vi "Camera Stream Properties.vi"() -> ()   [LabVIEW 2014]
doc: "When a camera stream is successfully opened, it is possible to edit its properties, like resolution and brightness.\nPlease note that the available properties are dependent on the camera type and driver."
uses:
  MSC Video_class/controls/Stream Property.ctl
  MSC Video_class/MSC Video.lvclass
  MSC Image_class/MSC Image.lvclass
panel:
  in  "Set":bool
  in  "New Value":dbl format="%#_3f"
  in  "Property":T1=3 caption="Camera Stream Property" items=["Position msec", "Position frames", "Position avi ratio", "Frame Width", "Frame Height", "FPS", "FourCC codec", "Frame Count", "Format", "Mode", "Brightness", "Contrast", "Saturation", "Hue", "Gain", "Exposure", "Convert RGB", "White Balance U", "Rectification", "Monochrome", "Sharpness", "Auto Exposure", "Gamma", "Temperature", "Trigger", "Trigger Delay", "White Balance V", "Zoom", "Focus", "Guid", "ISO Speed", "Max DV1394", "Backlight", "Pan", "Tilt", "Rolls", "Iris", "Settings", "Buffersize"]
  out "Properties":string[][](array[string])
  out "error out":errorcluster
  in  "stop":bool
  out "Live Image":picture
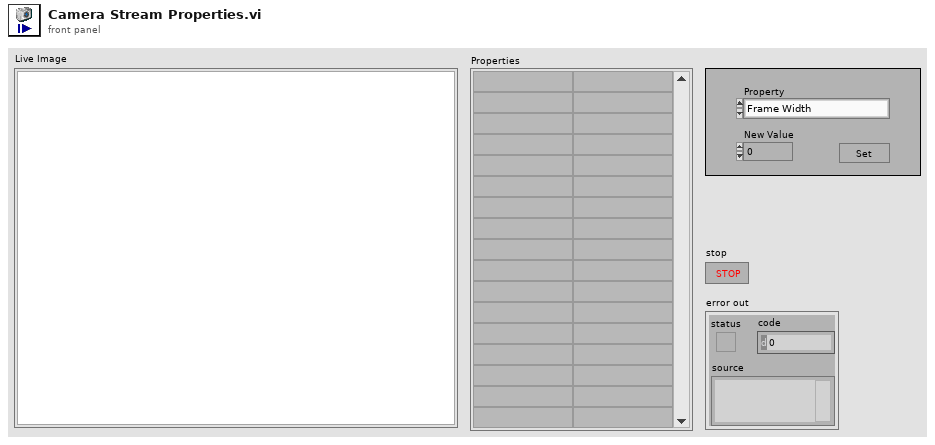
[diagram p1: front panel]
types:
  T1 = typedef "MSC Video.lvclass/Stream Property.ctl" = u16
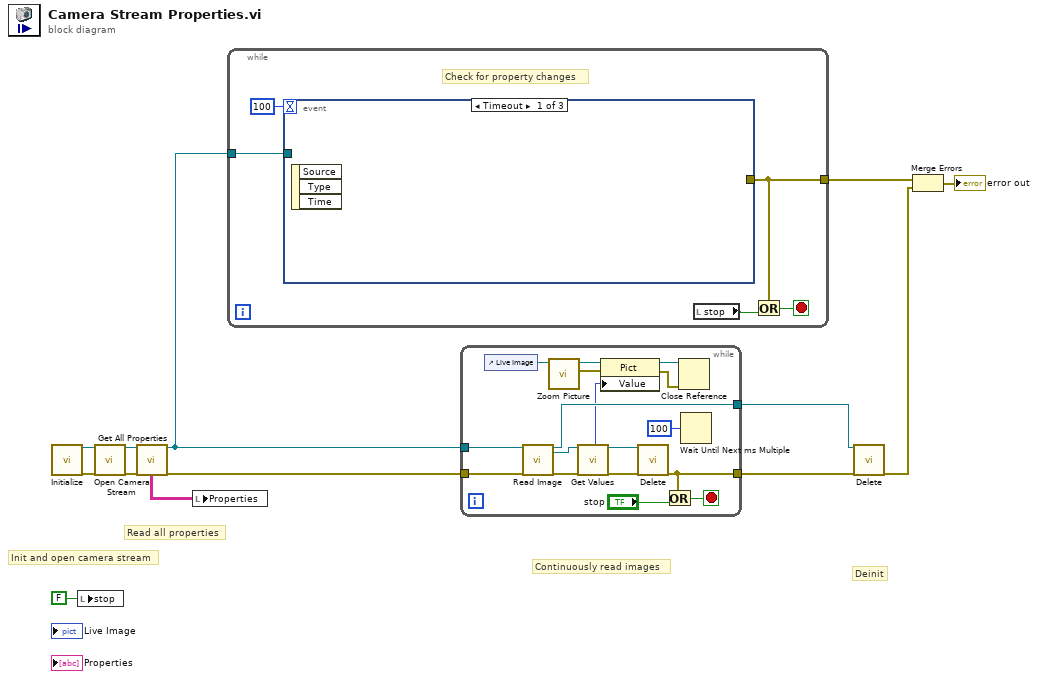
[diagram p0: block diagram]
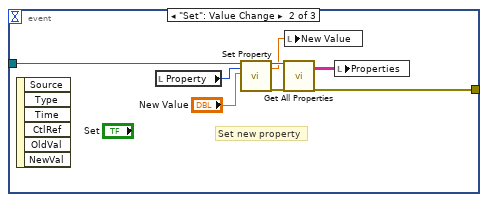
[diagram p2: hidden frame]
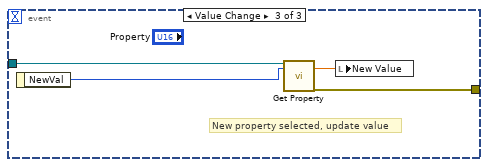
[diagram p3: hidden frame]
diagram:
  # "Deinit"
  # "Continuously read images"
  # "Read all properties"
  # "Init and open camera stream"
  n1 = call "Initialize.vi"() -> ("video out"=w13:refnum<class "MSC Video.lvclass">, "error out"=w12:errorcluster)  [unwired: 18 in]
  n2 = local write "stop"(FALSE ("stop")) -> ()
  n3 = call-dynamic "Open Camera Stream.vi"("video in"=w13, "error in (no error)"=w12) -> ("video out"=w9:refnum<class "MSC Video.lvclass">, "error out"=w8:errorcluster)  [unwired: 16 in]
  n4 = call-dynamic "Get All Properties.vi"("video in"=w9, "error in (no error)"=w8) -> ("video out"=w5:refnum<class "MSC Video.lvclass">, "Properties"=w6:string[][], "error out"=w7:errorcluster)  [unwired: 15 in]
  n5 = local write "Properties"(w6) -> ()
  n6 = while {
    tunnel: w5 -> [w18]
    tunnel: [w15] -> w2
    stop <- w16 stop-if-true
    # "Check for property changes"
    n7 = event shown="[0] Timeout" {
      selector: _ -> [_ _ _]
      dyn-events: _ -> [_ _ _]
      timeout: 100 -> [_ _ _]
      tunnel: w18 -> [_ w25 w28]
      tunnel: [_ w19 w27] -> w15
      event Timeout {
        n8 = event-data() -> ()  [unwired: 1 in, 3 out]
      }
      event "Set": Value Change {
        # "Set new property"
        n9 = event-data() -> ()  [unwired: 1 in, 6 out]
        n10 = local read "Property"() -> (w24:T1)
        n11 = call-dynamic "Set Property.vi"("video in"=w25, "Camera Stream Property"=w24, "propertyValue"="New Value") -> ("video out"=w22:refnum<class "MSC Video.lvclass">, "propertyValue out"=w20:dbl, "error out"=w21:errorcluster)  [unwired: 14 in]
        n12 = call-dynamic "Get All Properties.vi"("video in"=w22, "error in (no error)"=w21) -> ("Properties"=w23:string[][], "error out"=w19:errorcluster)  [unwired: 15 in, 1 out]
        n13 = local write "New Value"(w20) -> ()
        n14 = local write "Properties"(w23) -> ()
      }
      event Value Change {
        # "New property selected, update value"
        n15 = event-data() -> ("NewVal"=w29:T1)  [unwired: 1 in]
        n16 = call-dynamic "Get Property.vi"("video in"=w28, "Camera Stream Property"=w29) -> ("propertyValue"=w30:dbl, "error out"=w27:errorcluster)  [unwired: 15 in, 1 out]
        n17 = local write "New Value"(w30) -> ()
      }
    }
    n18 = local read "stop"() -> (w17:bool)
    n19 = Or(x=w15, y=w17) -> (x .or. y?=w16:bool)
  }
  n20 = while {
    tunnel: w5 -> [w47]
    tunnel: w7 -> [w46]
    tunnel: [w44] -> w11
    tunnel: [w38] -> w10
    stop <- w45 stop-if-true
    n21 = control-ref of="Live Image"() -> (w37:refnum<vi>)
    n22 = call-dynamic "Read Image.vi"("video in"=w47, "error in (no error)"=w46) -> ("video out"=w44:refnum<class "MSC Video.lvclass">, "image out"=w43:refnum<class "MSC Image.lvclass">, "error out"=w42:errorcluster)  [unwired: 15 in]
    n23 = call "Zoom Picture.vi"("Picture in"=w37) -> ("error out"=w35:errorcluster, "Picture out"=w36:refnum<vi>)  [unwired: 9 in]
    n24 = call-dynamic "Get Values.vi"("image in"=w43, "error in (no error)"=w42) -> ("picture"=w34:picture, "image out"=w40:refnum<class "MSC Image.lvclass">, "error out"=w39:errorcluster)  [unwired: 10 in, 5 out]
    n25 = property class="Pict"(reference=w36, error in=w35, "Value"=w34) -> (reference out=w33:refnum<vi>, error out=w32:errorcluster)
    n26 = call-dynamic "Delete.vi"("image in"=w40, "error in (no error)"=w39) -> ("error out"=w38:errorcluster)  [unwired: 17 in]
    n27 = Or(x=w38, y="stop") -> (x .or. y?=w45:bool)
    n28 = Close Reference(reference=w33, error in (no error)=w32) -> ()  [unwired: 1 out]
    n29 = Wait Until Next ms Multiple(millisecond multiple=u32 100) -> ()  [unwired: 1 out]
  }
  n30 = call-dynamic "Delete.vi"("video in"=w11, "error in (no error)"=w10) -> ("error out"=w1:errorcluster)  [unwired: 17 in]
  n31 = Merge Errors(w2, w1) -> (→"error out":errorcluster)
